vi "Draw Graph.vi"(7 "History Graph State in":T1, 8 "error in (no error)":errorcluster, 9 "Scrollbar in":u64(c297), 10 "Live Button":bool) -> (0 "error out":errorcluster, 1 "Scrollbar out":u64, 2 "Waveform Graph":waveform(dbl)[](graph), 4 "Number of values in file":u64, 5 "History Graph State out":T1)   [LabVIEW 2021, in "History Graph.lvlib"]
uses:
  History Graph.lvlib
  Controls/History Graph State Cluster.ctl
panel:
  out "group/channel names":string[][](array[string])
  out "group names":string[](array[string])
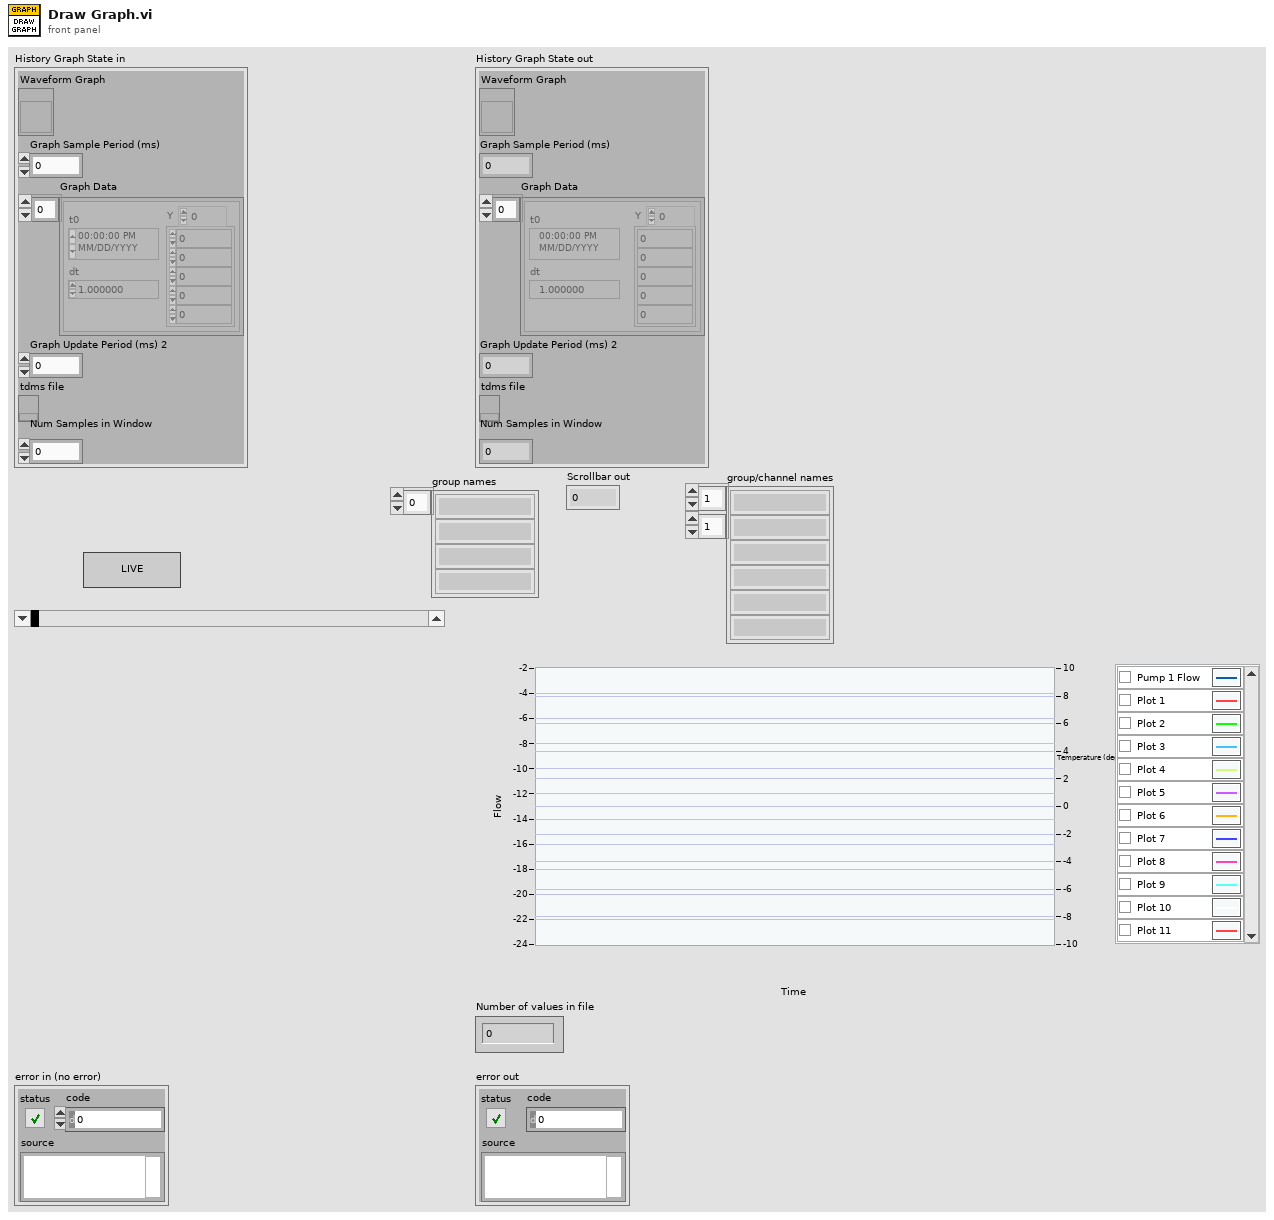
[diagram p1: front panel]
types:
  T1 = typedef "History Graph.lvlib/History Graph State Cluster.ctl" = cluster{"Waveform Graph":refnum<vi>, "Graph Sample Period (ms)":i32, "Graph Data":waveform(dbl)[], "Graph Update Period (ms) 2":i32, "tdms file":refnum<k34>, "Num Samples in Window":i64}
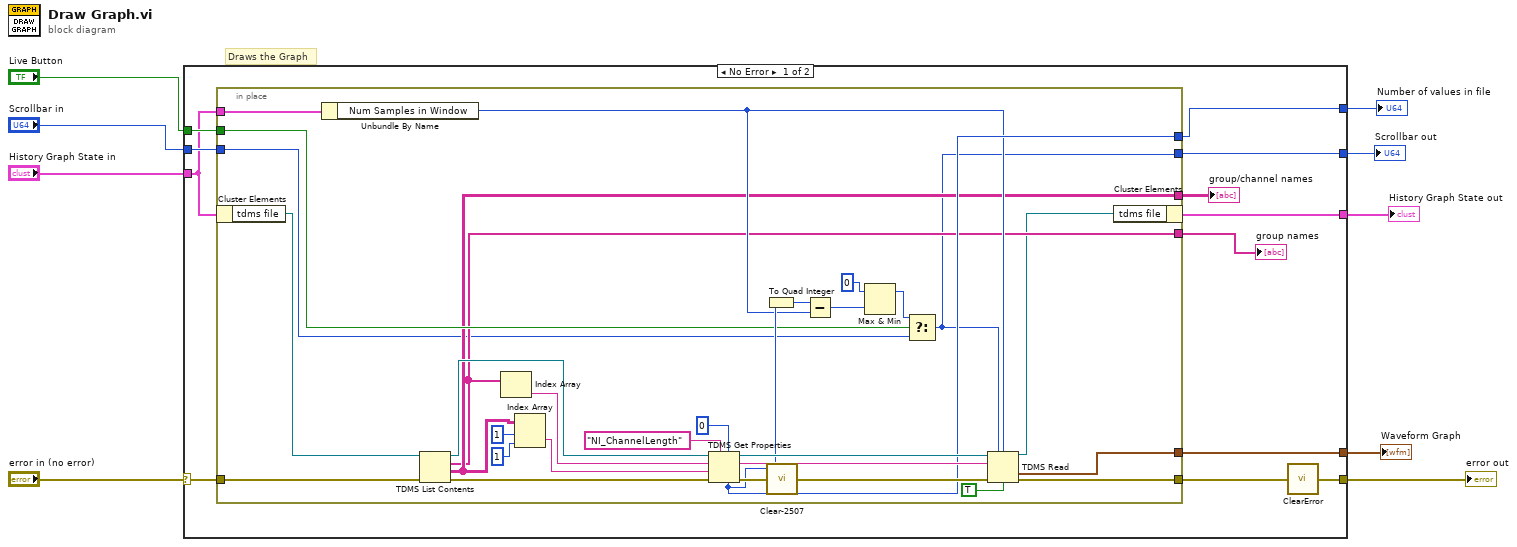
[diagram p0: block diagram]
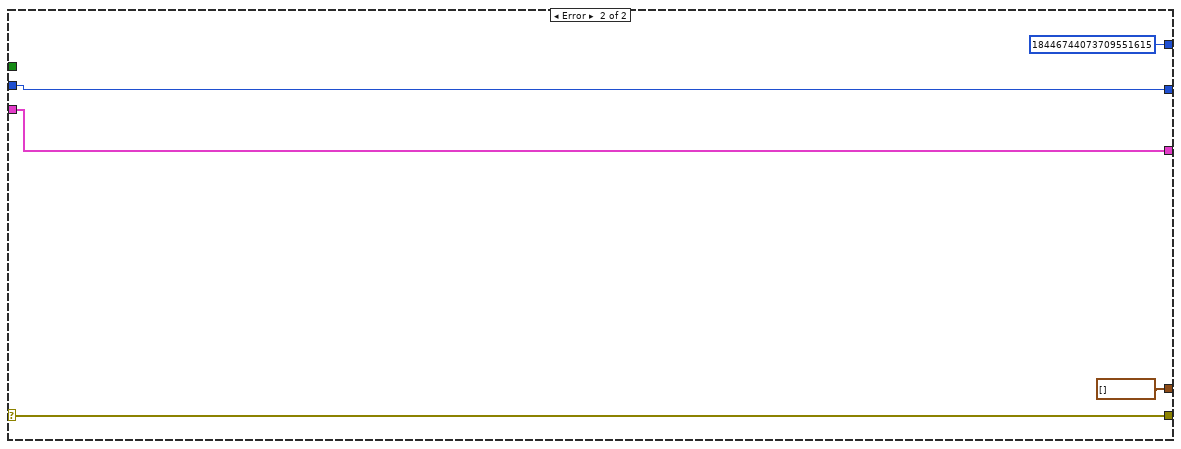
[diagram p2: hidden frame]
diagram:
  # "Draws the Graph"
  n1 = case shown="No Error" "error in (no error)" {
    selector: "error in (no error)" -> [w18 w55]
    tunnel: [w19 w55] -> w7
    tunnel: "History Graph State in" -> [w13 w56]
    tunnel: [w12 w56] -> w9
    tunnel: "Live Button" -> [w21 _]
    tunnel: [w15 w54] -> w4
    tunnel: "Scrollbar in" -> [w14 w54]
    tunnel: [w11 u64 18446744073709551615] -> w2
    tunnel: [w10 waveform(dbl)[] []] -> w1
    frame No Error {
      n2 = in-place {
        in-place-border: [w45] -> w11
        in-place-border: w21 -> [w41]
        in-place-border: [w40] -> w20
        in-place-border: w13 -> [w37]
        in-place-border: [w36] -> w10
        in-place-border: w18 -> [w34]
        in-place-border: [w32] -> w17
        in-place-border: [w29] -> w16
        in-place-border: [w26] -> w15
        in-place-border: w14 -> [w25]
        n3 = in-place-cluster #1(w13) -> ("tdms file"=w23:refnum<k34>)
        n4 = Unbundle By Name(w37) -> ("Num Samples in Window"=w38:i64)
        n5 = TDMS List Contents(4:w34, 7:w23) -> (0:w33:errorcluster, 1:w32:string[][], 2:w29:string[], 3:w35:refnum<k34>)  [unwired: 1 in]
        n6 = Index Array(array=w29) -> (element=w28:string)  [unwired: 1 in]
        n7 = Index Array(array=w32, index (row)=1, index (col)=1 ("disabled index (col)")) -> (element=w24:string)
        n8 = TDMS Get Properties(5:u64 0, 7:"NI_ChannelLength" ("channel name(s) in"), 8:w33, 9:w24, 10:w28, 11:w35) -> (0:w47:errorcluster, 2:w48:string, 3:w49:refnum<k34>, 4:w45:u64)  [unwired: 2 out]
        n9 = To Quad Integer(1:w45) -> (0:w27:i64)
        n10 = call <vilib>:"Clear-2507.vi"("error in (no error)"=w47) -> ("error out"=w46:errorcluster)
        n11 = Subtract(x=w27, y=w38) -> (x-y=w43:i64)
        n12 = Max & Min(x=i64 0, y=w43) -> (max(x,y)=w42:i64)  [unwired: 1 out]
        n13 = Select(t=w42, s=w41, f=w25) -> (s? t:f=w26:u64)
        n14 = TDMS Read(0:w49, 1:w26, 2:w38, 5:w48, 11:w46, 13:TRUE ("return channels in file order? (F)")) -> (4:w22:refnum<k34>, 10:w36:waveform(dbl)[], 15:w40:errorcluster)  [unwired: 2 in, 3 out]
        n15 = in-place-cluster #1("tdms file"=w22) -> (w12:T1)
      }
      "group names" <- w16
      "group/channel names" <- w17
      n16 = call <vilib>:"ClearError.vi"("error in (no error)"=w20) -> ("error out"=w19:errorcluster)
    }
    frame Error {
    }
  }
  "History Graph State out" <- w9
  "error out" <- w7
  "Scrollbar out" <- w4
  "Number of values in file" <- w2
  "Waveform Graph" <- w1
